vi "Get Enqueuer.vi"(8 "error in (no error)":errorcluster, 11 "[V] Tester Parent in":refnum<class "[V] Tester Parent.lvclass">) -> (0 "error out":errorcluster, 3 "[V] Tester Parent out":refnum<class "[V] Tester Parent.lvclass">)   [LabVIEW 2020, in "[V] Tester Parent.lvlib" / "[V] Tester Parent.lvclass"]
uses:
  [V] Tester Parent.lvclass
  C:/Program Files (x86)/National Instruments/LabVIEW 2020/vi.lib/ActorFramework/Actor/Actor.lvclass
  <vilib>/ActorFramework/Actor/Actor.lvclass/Actor.ctl
  <vilib>/ActorFramework/Message Enqueuer/Message Enqueuer.lvclass/Message Enqueuer.ctl
  [V] Tester Parent.lvclass/[V] Tester Parent.ctl
  <vilib>/ActorFramework/Message Enqueuer/Init from Existing Queue.vi
  <vilib>/ActorFramework/Message Enqueuer/Message Enqueuer.lvclass
  <vilib>/ActorFramework/Actor/Actor.lvclass
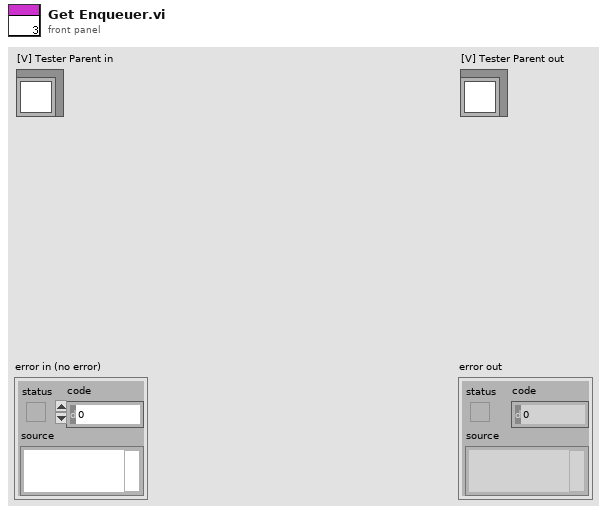
[diagram p1: front panel]
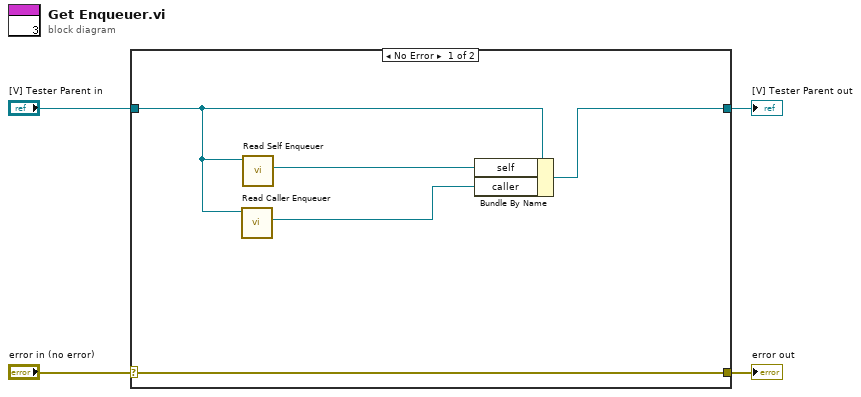
[diagram p0: block diagram]
diagram:
  n1 = case shown="No Error" "error in (no error)" {
    selector: "error in (no error)" -> [w9 w11]
    tunnel: [w9 w11] -> w3
    tunnel: [w5 w10] -> w1
    tunnel: "[V] Tester Parent in" -> [w8 w10]
    frame No Error {
      n2 = call <vilib>:"Read Caller Enqueuer.vi"("Actor"=w8) -> ("Caller Enqueuer"=w6:refnum<class "Message Enqueuer.lvclass">)  [unwired: 10 in]
      n3 = call <vilib>:"Read Self Enqueuer.vi"("Actor"=w8) -> ("Self Enqueuer"=w7:refnum<class "Message Enqueuer.lvclass">)  [unwired: 10 in]
      n4 = Bundle By Name(cluster=w8, "self"=w7, "caller"=w6) -> (w5:refnum<class "[V] Tester Parent.lvclass">)
    }
    frame Error {
    }
  }
  "error out" <- w3
  "[V] Tester Parent out" <- w1
